vi "Create.vi"(8 "error in (no error)":errorcluster, 11 "DBL array in":dbl[](array[numeric])) -> (0 "error out":errorcluster, 3 "Float64Array out":refnum<class "Float64Array.lvclass">)   [LabVIEW 2013, in "MDSplus.lvlib" / "Float64Array.lvclass"]
uses:
  <vilib>/MDSplus/Classes/Data_Class/Array_Class/Float64Array_Class/Float64Array.lvclass
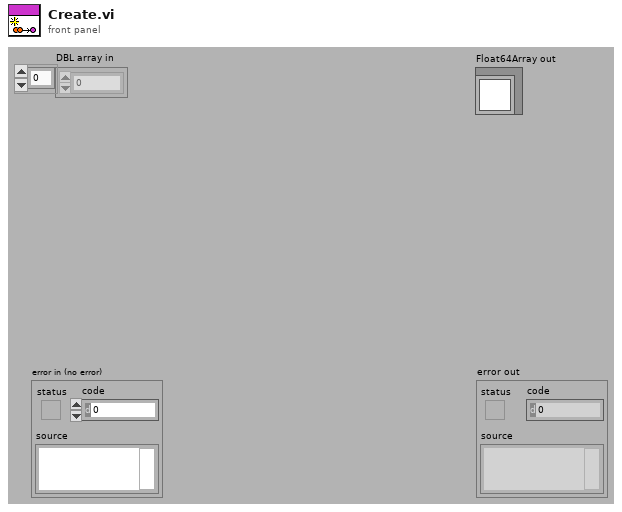
[diagram p1: front panel]
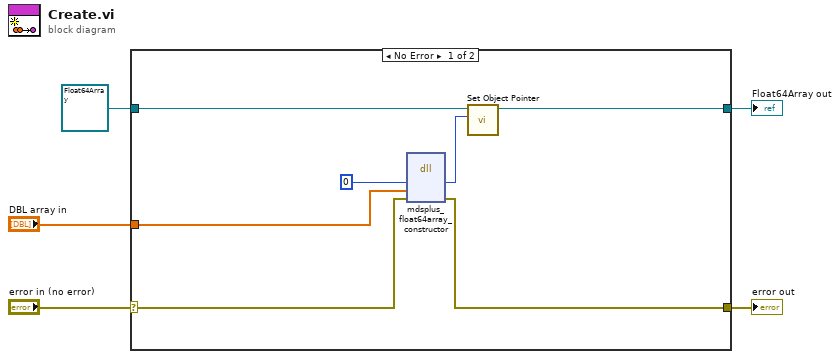
[diagram p0: block diagram]
diagram:
  n1 = case shown="No Error" "error in (no error)" {
    selector: "error in (no error)" -> [w10 w14]
    tunnel: [w6 w14] -> w4
    tunnel: [w8 w13] -> w2
    tunnel: refnum<class "Float64Array.lvclass"> refnum ("Float32 in") -> [w9 w13]
    tunnel: "DBL array in" -> [w7 _]
    frame No Error {
      n2 = dll-call lib="MDSobjectsLVShr" fn="mdsplus_float64array_constructor"("lvFloat64ArrayPtrOut"=i64 0 ("lvTreePtr"), "lvDblArrHdlIn"=w7, "error"=w10) -> ("lvFloat64ArrayPtrOut"=w11:i64, "error"=w6:errorcluster)  [unwired: 5 in, 2 out]
      n3 = call-dynamic "Set Object Pointer.vi"("Object Pointer"=w11, "Data in"=w9) -> ("Data out"=w8:refnum<class "Float64Array.lvclass">)  [unwired: 9 in]
    }
    frame Error {
    }
  }
  "error out" <- w4
  "Float64Array out" <- w2
